vi "BRig_RT__Case_Exp__State_CuePre__v5.vi"(0 "input_dataCurrent":u16[](array[numeric]), 1 "input_dataTrial":u16[][](array[numeric]), 2 "input_dataExp":u16[](array[numeric]), 3 "input_Cue2":bool, 6 "input_I_lick":bool, 9 "input_arrTrig":bool[](array[boolean])) -> (12 "output_state":T1, 13 "output_arrTrig":bool[](array[boolean]), 14 "output_dataCurrent":u16[](array[numeric]), 15 "output_dataTrial":u16[][](array[numeric]))   [LabVIEW 2014]
uses:
  myRIO_BRig_RT__Case_Exp_stateList.ctl
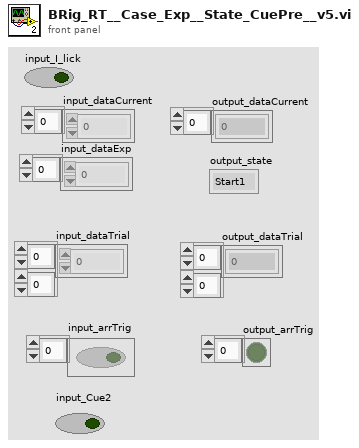
[diagram p1: front panel]
types:
  T1 = typedef "myRIO_BRig_RT__Case_Exp_stateList.ctl" = enum16{"Start1", "Start2", "Start3", "saveSettings1", "saveSettings2", "saveSettings3", "saveSettings4", "saveSettings_LC_ENL_l1", "saveSettings_LC_ENL_l2", "saveSettings_LC_Cue_l1", "saveSettings_LC_Cue_l2", "saveSettings6_LC_l1_Other", "SaveSettings6_LC_l2_Other", "setSettings_Audio", "setSettings_Laser", "initBlock_pre", "initBlock", "initBlock2", "initBlock_post", "initTrial_pre", "initTrial", "initTrial2", "initTrial3", "initTrial4", "initTrial_LC_ENL1", "initTrial_LC_Cue1", "initTrial_LC_Cue1_2", "initTrial_LC_Sel", "initTrial_post", "ENL1_pre", "ENL1", "ENL1_post", "ENL1Penalty_pre", "ENL1Penalty", "ENL2_pre", "ENL2", "ENL2Penalty_pre", "ENL2Penalty", "Cue1_pre", "Cue1", "Cue1_post", "Cue1Penalty_pre", "Cue1Penalty", "Cue2_pre", "Cue2", "Cue2Penalty_pre", "Cue2Penalty", "Selection_pre", "Selection", "Select_post", "SelectReward_pre", "SelectReward", "SelectRewardPost_pre", "SelectRewardPost", "SelectWrong_pre", "SelectWrong", "SelectWrong_post", "SelectTimeout_pre", "SelectTimeout", "SelectTimeout_post", "endTrial_pre", "endTrial1", "endTrial2", "endTrial3", "endTrial_post", "endBlock_pre", "endBlock", "endBlock_post", "endExp", "commConnect", "commUpload_pre", "commUpload_dataBlock", "commUpload_dataCurrent", "commUpload_dataExp", "commUpload_dataLC", "commUpload_dataTrial", "commUpload_post", "saveData_pre", "saveData_dataBlock", "saveData_dataCurrent", "saveData_dataExp", "saveData_dataLC", "saveData_dataTrial", "saveData_post", "empty_endBlock1", "empty_endBlock2", "empty_endTrial1", "empty_endTrial2", "empty_endTrial3", "empty_endTrial4", "empty_endTrial5", "dummyState", "dummyState_endBlock", "FreeReward_pre", "FreeReward", "FreeRewardPost_pre", "FreeRewardPost"}
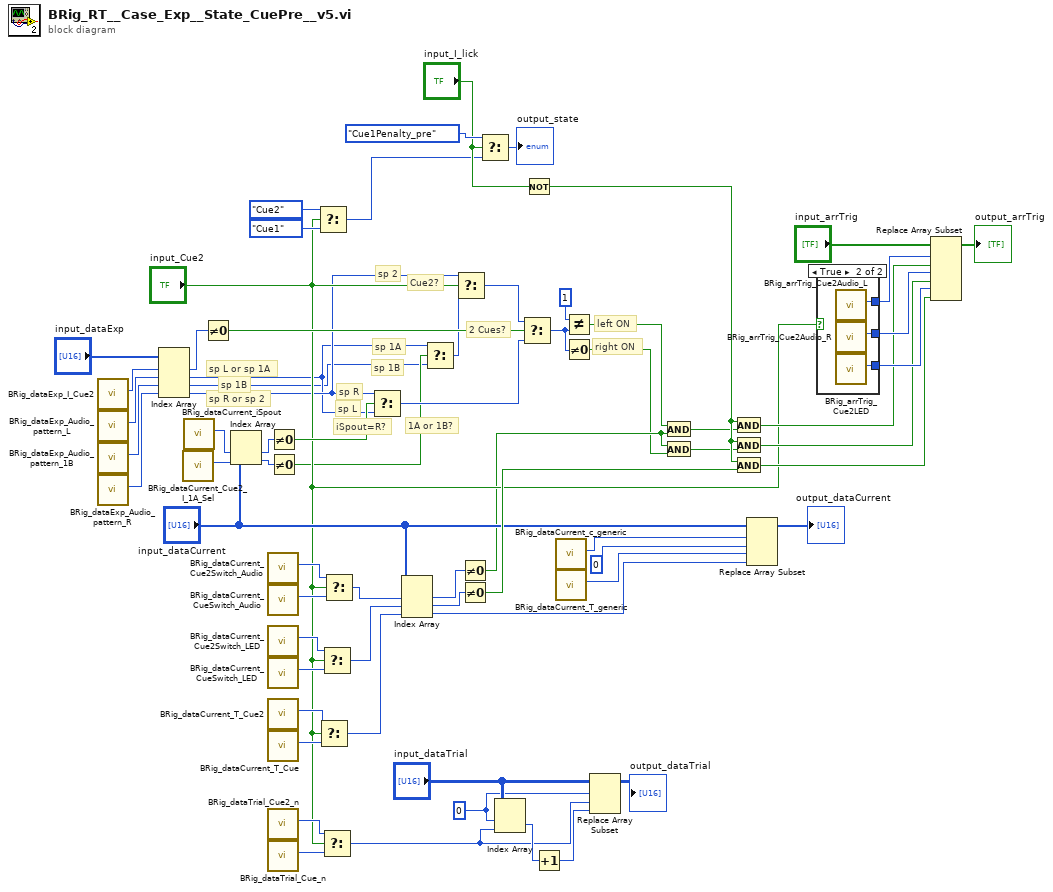
[diagram p0: block diagram]
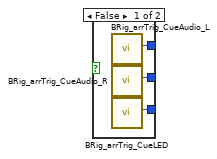
[diagram p2: hidden frame]
diagram:
  w44 = 0
  # "right ON"
  # "left ON"
  # "2 Cues?"
  # "sp 1A"
  # "1A or 1B?"
  # "sp 1B"
  # "sp 1B"
  # "sp L or sp 1A"
  # "sp R or sp 2"
  # "sp 2"
  # "Cue2?"
  # "sp R"
  # "sp L"
  # "iSpout=R?"
  n1 = call "BRig_dataExp_I_Cue2.vi"() -> ("output_I_Cue2"=w25:i32)  [unwired: 11 in]
  n2 = call "BRig_dataExp_Audio_pattern_L.vi"() -> ("output_Audio_sp__L"=w24:i32)  [unwired: 11 in]
  n3 = call "BRig_dataExp_Audio_pattern_1B.vi"() -> ("output_Audio_sp__1B"=w23:i32)  [unwired: 11 in]
  n4 = call "BRig_dataExp_Audio_pattern_R.vi"() -> ("output_Audio_sp__R"=w22:i32)  [unwired: 11 in]
  n5 = Index Array(array="input_dataExp", index #1=w25, index #2=w24, index #3=w23, index #4=w22) -> (element #1=w20:u16, element #2=w11:u16, element #3=w10:u16, element #4=w13:u16)
  n6 = call "BRig_dataCurrent_Cue2_I_1A_Sel.vi"() -> ("output_Cue2_I_1A_Sel"=w26:i32)  [unwired: 11 in]
  n7 = call "BRig_dataCurrent_iSpout.vi"() -> ("output_iSpout"=w21:i32)  [unwired: 11 in]
  n8 = Not Equal To 0?(x=w20) -> (x != 0?=w17:bool)
  n9 = Index Array(array="input_dataCurrent", index #1=w21, index #2=w26) -> (element #1=w18:u16, element #2=w19:u16)
  n10 = call "BRig_dataCurrent_Cue2Switch_Audio.vi"() -> ("output_Cue2Switch_Audio"=w30:i32)  [unwired: 11 in]
  n11 = call "BRig_dataCurrent_CueSwitch_Audio.vi"() -> ("output_CueSwitch_Audio"=w31:i32)  [unwired: 11 in]
  n12 = call "BRig_dataCurrent_Cue2Switch_LED.vi"() -> ("output_Cue2Switch_LED"=w34:i32)  [unwired: 11 in]
  n13 = call "BRig_dataCurrent_CueSwitch_LED.vi"() -> ("output_CueSwitch_LED"=w33:i32)  [unwired: 11 in]
  n14 = call "BRig_dataCurrent_T_Cue2.vi"() -> ("output_T_Cue2"=w39:i32)  [unwired: 11 in]
  n15 = call "BRig_dataCurrent_T_Cue.vi"() -> ("output_T_Cue"=w40:i32)  [unwired: 11 in]
  n16 = call "BRig_dataTrial_Cue2_n.vi"() -> ("output_Cue2_n"=w36:i32)  [unwired: 11 in]
  n17 = call "BRig_dataTrial_Cue_n.vi"() -> ("output_Cue_n"=w37:i32)  [unwired: 11 in]
  n18 = Not Equal To 0?(x=w18) -> (x != 0?=w16:bool)
  n19 = Not Equal To 0?(x=w19) -> (x != 0?=w12:bool)
  n20 = Select(t=myRIO_BRig_RT__Case_Exp_stateList."Cue2", s="input_Cue2", f=myRIO_BRig_RT__Case_Exp_stateList."Cue1" ("Enum")) -> (s? t:f=w42:T1)
  n21 = Select(t=w39, s="input_Cue2", f=w40) -> (s? t:f=w38:i32)
  n22 = Select(t=w34, s="input_Cue2", f=w33) -> (s? t:f=w32:i32)
  n23 = Select(t=w36, s="input_Cue2", f=w37) -> (s? t:f=w35:i32)
  n24 = Select(t=w30, s="input_Cue2", f=w31) -> (s? t:f=w29:i32)
  n25 = Select(t=w13, s=w16, f=w11) -> (s? t:f=w15:u16)
  n26 = Index Array(array="input_dataCurrent", index #1=w29, index #2=w32, index #3=w38) -> (element #1=w61:u16, element #2=w60:u16, element #3=w62:u16)
  n27 = Select(t=w11, s=w12, f=w10) -> (s? t:f=w9:u16)
  n28 = Select(t=w13, s="input_Cue2", f=w9) -> (s? t:f=w8:u16)
  n29 = Not Equal To 0?(x=w61) -> (x != 0?=w3:bool)
  n30 = Not Equal To 0?(x=w60) -> (x != 0?=w58:bool)
  n31 = Select(t=myRIO_BRig_RT__Case_Exp_stateList."Cue1Penalty_pre" ("Enum"), s="input_I_lick", f=w42) -> (s? t:f=→"output_state":T1)
  n32 = Index Array(array="input_dataTrial", index (row)=w44, index (col)=w35) -> (element=w55:u16)
  n33 = Select(t=w8, s=w17, f=w15) -> (s? t:f=w6:u16)
  n34 = Not(x="input_I_lick") -> (.not. x?=w57:bool)
  n35 = Increment(x=w55) -> (x+1=w54:u16)
  n36 = call "BRig_dataCurrent_c_generic.vi"() -> ("output_count_generic"=w65:i32)  [unwired: 11 in]
  n37 = call "BRig_dataCurrent_T_generic.vi"() -> ("output_T_generic"=w64:i32)  [unwired: 11 in]
  n38 = Not Equal?(x=u16 1 ("y"), y=w6) -> (x != y?=w2:bool)
  n39 = Not Equal To 0?(x=w6) -> (x != 0?=w1:bool)
  n40 = Replace Array Subset(array="input_dataTrial", new element=w54, index (row)=w44, index (col)=w35) -> (→"output_dataTrial":u16[][])
  n41 = And(x=w2, y=w3) -> (x .and. y?=w5:bool)
  n42 = And(x=w3, y=w1) -> (x .and. y?=w4:bool)
  n43 = And(x=w57, y=w5) -> (x .and. y?=w46:bool)
  n44 = And(x=w57, y=w4) -> (x .and. y?=w47:bool)
  n45 = And(x=w57, y=w58) -> (x .and. y?=w48:bool)
  n46 = Replace Array Subset(array="input_dataCurrent", new element #1=u16 0 ("new element/subarray"), index #1=w65, new element #2=w62, index #2=w64) -> (→"output_dataCurrent":u16[])
  n47 = case shown="True" "input_Cue2" {
    tunnel: [w71 w74] -> w51
    tunnel: [w70 w73] -> w50
    tunnel: [w69 w72] -> w49
    frame False {
      n48 = call "BRig_arrTrig_CueAudio_L.vi"() -> ("output_CueAudio_L"=w71:i32)  [unwired: 11 in]
      n49 = call "BRig_arrTrig_CueAudio_R.vi"() -> ("output_CueAudio_R"=w70:i32)  [unwired: 11 in]
      n50 = call "BRig_arrTrig_CueLED.vi"() -> ("output_CueLED"=w69:i32)  [unwired: 11 in]
    }
    frame True {
      n51 = call "BRig_arrTrig_Cue2Audio_L.vi"() -> ("output_Cue2Audio_L"=w74:i32)  [unwired: 11 in]
      n52 = call "BRig_arrTrig_Cue2Audio_R.vi"() -> ("output_Cue2Audio_R"=w73:i32)  [unwired: 11 in]
      n53 = call "BRig_arrTrig_Cue2LED.vi"() -> ("output_Cue2LED"=w72:i32)  [unwired: 11 in]
    }
  }
  n54 = Replace Array Subset(array="input_arrTrig", new element #1=w46, index #1=w51, new element #2=w47, index #2=w50, new element #3=w48, index #3=w49) -> (→"output_arrTrig":bool[])
